vi "CreateListener.vi"(8 "error in (no error)":errorcluster, 11 "TCP_Listener in":refnum<class "TCP_Listener.lvclass">) -> (0 "error out":errorcluster, 3 "TCP_Listener out":refnum<class "TCP_Listener.lvclass">)   [LabVIEW 2023, in "TCP_Listener.lvlib" / "TCP_Listener.lvclass"]
uses:
  TCP_Listener.lvclass
  C:/Program Files (x86)/National Instruments/LabVIEW 2023/vi.lib/ActorFramework/Actor/Actor.lvclass
  <vilib>/ActorFramework/Actor/Actor.lvclass/Actor.ctl
  <vilib>/ActorFramework/Message Enqueuer/Message Enqueuer.lvclass/Message Enqueuer.ctl
  TCP_Listener.lvclass/TCP_Listener.ctl
  <vilib>/ActorFramework/Message Enqueuer/Init from Existing Queue.vi
  <vilib>/ActorFramework/Message Enqueuer/Enqueue.vi
  TCP_Listener Messages/Listen Msg/Listen Msg.lvclass
  C:/Program Files (x86)/National Instruments/LabVIEW 2023/vi.lib/ActorFramework/Message/Message.lvclass
  <vilib>/ActorFramework/Stop Msg/Stop Msg.lvclass
  TCP_Listener Messages/CreateListener Msg/CreateListener Msg.lvclass
  <vilib>/ActorFramework/Message Priority Queue/Priority Enqueue.vi
  <vilib>/ActorFramework/Message Enqueuer/Message Enqueuer.lvclass
  <vilib>/ActorFramework/Actor/Actor.lvclass
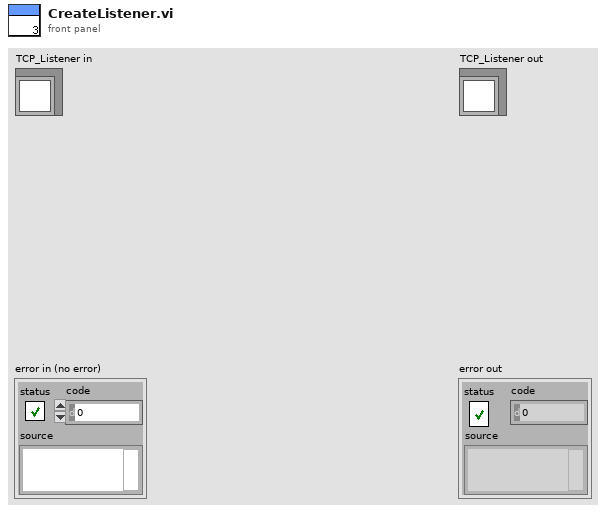
[diagram p1: front panel]
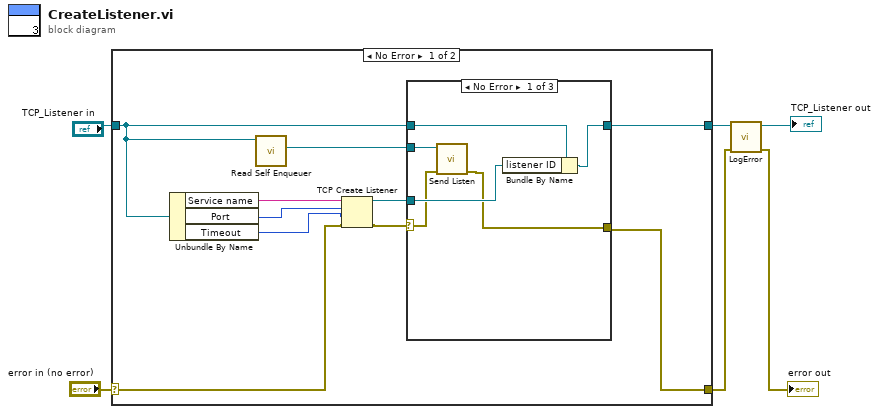
[diagram p0: block diagram]
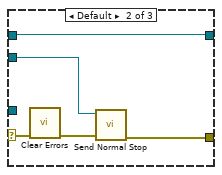
[diagram p2: hidden frame]
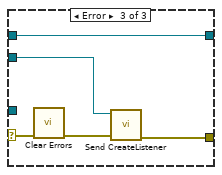
[diagram p3: hidden frame]
diagram:
  n1 = case shown="No Error" "error in (no error)" {
    selector: "error in (no error)" -> [w14 w34]
    tunnel: [w9 w34] -> w2
    tunnel: [w10 w33] -> w4
    tunnel: "TCP_Listener in" -> [w13 w33]
    frame No Error {
      n2 = Unbundle By Name(w13) -> ("Service name"=w16:string, "Port"=w7:u16, "Timeout"=w15:i32)
      n3 = call <vilib>:"Read Self Enqueuer.vi"("Actor"=w13) -> ("Self Enqueuer"=w8:refnum<class "Message Enqueuer.lvclass">)  [unwired: 10 in]
      n4 = TCP Create Listener(8:w14, 9:w15, 10:w7, 11:w16) -> (0:w12:errorcluster, 3:w11:refnum<k5>)  [unwired: 1 in, 1 out]
      n5 = case shown="No Error" w12 {
        selector: w12 -> [w18 w24 w29]
        tunnel: w13 -> [w22 w27 w32]
        tunnel: w11 -> [w21 _ _]
        tunnel: [w20 w27 w32] -> w10
        tunnel: [w17 w26 w30] -> w9
        tunnel: w8 -> [w19 w25 w31]
        frame No Error {
          n6 = call "Send Listen.vi"("error in (no error)"=w18, "Message Enqueuer"=w19) -> ("error out"=w17:errorcluster)  [unwired: 8 in, 1 out]
          n7 = Bundle By Name(cluster=w22, "listener ID"=w21) -> (w20:refnum<class "TCP_Listener.lvclass">)
        }
        frame Default {
          n8 = call <vilib>:"Clear Errors.vi"("error in (no error)"=w24) -> ("error out"=w23:errorcluster)  [unwired: 5 in, 1 out]
          n9 = call <vilib>:"Send Normal Stop.vi"("error in (no error)"=w23, "Message Enqueuer"=w25) -> ("error out"=w26:errorcluster)  [unwired: 9 in]
        }
        frame Error {
          n10 = call <vilib>:"Clear Errors.vi"("error in (no error)"=w29) -> ("error out"=w28:errorcluster)  [unwired: 5 in, 1 out]
          n11 = call "Send CreateListener.vi"("error in (no error)"=w28, "Message Enqueuer"=w31) -> ("error out"=w30:errorcluster)  [unwired: 8 in, 1 out]
        }
      }
    }
    frame Error {
    }
  }
  n12 = call "LogError.vi"("error in (no error)"=w2, "TCP_Listener in"=w4) -> ("error out"=→"error out":errorcluster, "TCP_Listener out"=→"TCP_Listener out":refnum<class "TCP_Listener.lvclass">)  [unwired: 8 in]
